vi "ObjectAvoid.vi"(7 "Stop?":bool, 8 "error in (no error)":errorcluster, 11 "RobotDriveDevRef":T1) -> (2 "Motor Values":dbl[](array[numeric]))   [LabVIEW 2015]
uses:
  <vilib>/Rock Robotics/WPI/RobotDrive/WPI_RobotDriveDevRef.ctl
  <vilib>/Rock Robotics/WPI/MotorControl/WPI_MotorControlDeviceRef.ctl
  <vilib>/Rock Robotics/WPI/MotorControl/WPI_MotorControlType.ctl
  <vilib>/Rock Robotics/SystemInterfaces/DIO/FPGA_DIOPWMChannel.ctl
  <vilib>/Rock Robotics/WPI/PWM/WPI_PWMDeadband.ctl
  <vilib>/Rock Robotics/WPI/CAN/Jaguar/SubVIs/WPI_CANJaguar_ControlMode.ctl
  <vilib>/Rock Robotics/WPI/CAN/TalonSRX/WPI_CANTalonSRX_APIControlMode.ctl
  Robot Global Data.vi
  <vilib>/Rock Robotics/WPI/RobotDrive/WPI_RobotDriveArcadeDrive_Standard(NoSaturation).vi
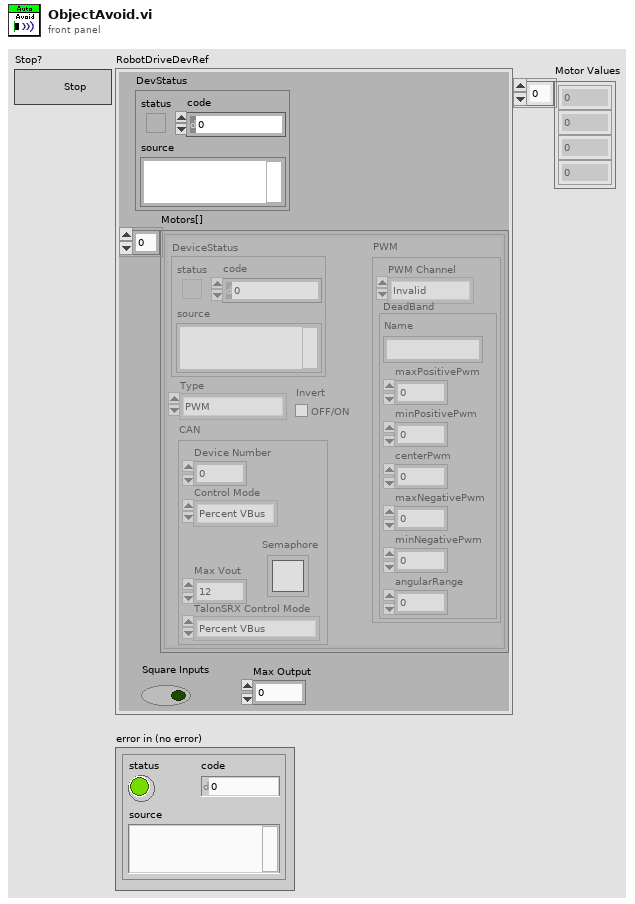
[diagram p1: front panel]
types:
  T1 = typedef "WPI_RobotDriveDevRef.ctl" = cluster{"DevStatus":errorcluster, "Motors[]":T2[], "Square Inputs":bool, "Max Output":dbl}
  T2 = typedef "WPI_MotorControlDeviceRef.ctl" = cluster{"DeviceStatus":errorcluster, "Type":T3, "PWM":cluster{"PWM Channel":T4, "DeadBand":T5}, "CAN":cluster{"Device Number":u8, "Control Mode":T6, "Semaphore":T7, "Max Vout":dbl, "TalonSRX Control Mode":T8}, "Invert":bool}
  T3 = typedef "WPI_MotorControlType.ctl" = enum16{"PWM", "CAN", "CANTalonSRX"}
  T4 = typedef "FPGA_DIOPWMChannel.ctl" = enum8{"PWM 0", "PWM 1", "PWM 2", "PWM 3", "PWM 4", "PWM 5", "PWM 6", "PWM 7", "PWM 8", "PWM 9", "PWM MXP 0", "PWM MXP 1", "PWM MXP 2", "PWM MXP 3", "PWM MXP 4", "PWM MXP 5", "PWM MXP 6", "PWM MXP 7", "PWM MXP 8", "PWM MXP 9", "Invalid"}
  T5 = typedef "WPI_PWMDeadband.ctl" = cluster{"Name":string, "maxPositivePwm":i32, "minPositivePwm":i32, "centerPwm":i32, "maxNegativePwm":i32, "minNegativePwm":i32, "angularRange":u16}
  T6 = typedef "WPI_CANJaguar_ControlMode.ctl" = enum8{"Percent VBus", "Current", "Speed", "Position", "Voltage"}
  T7 = typedef "Semaphore RefNum" = refnum<k1>
  T8 = typedef "WPI_CANTalonSRX_APIControlMode.ctl" = enum8{"Percent VBus", "Speed", "Position", "Slave", "Unchanged / Invalid", "Voltage Compensation", "Current", "Motion Profile"}
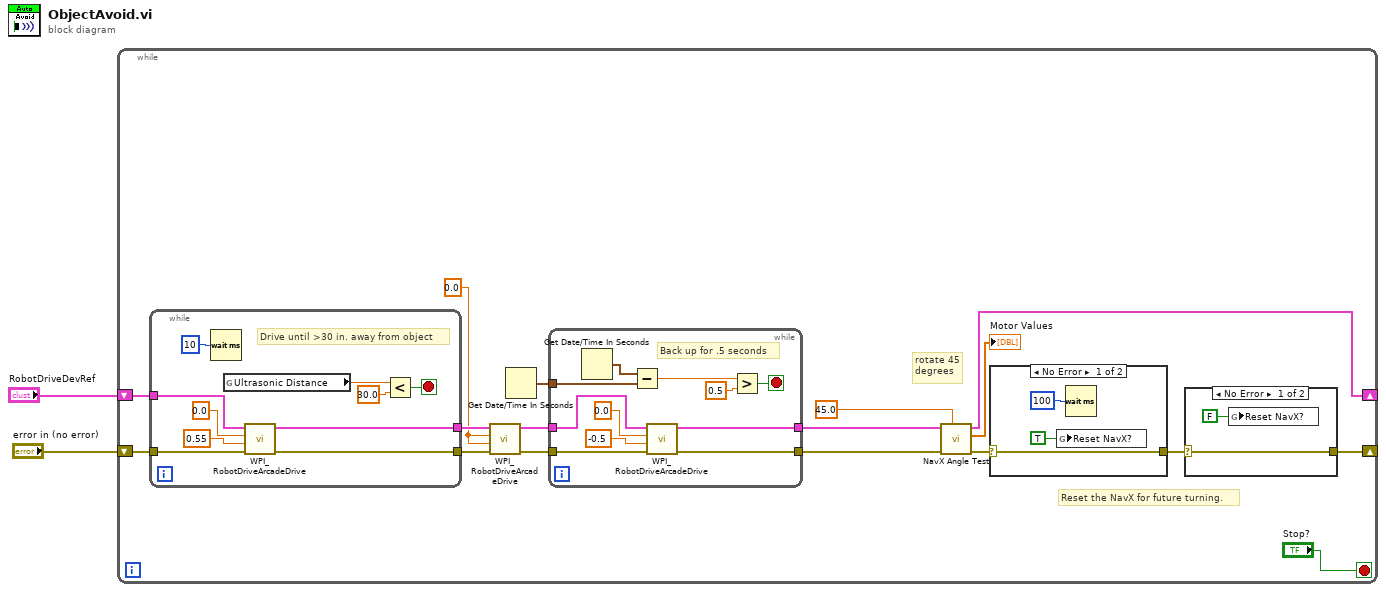
[diagram p0: block diagram]
diagram:
  n1 = while {
    shift-right: [w10] -> _
    shift-left: "RobotDriveDevRef" -> [w13]
    shift-right: [w6] -> _
    shift-left: "error in (no error)" -> [w5]
    stop <- "Stop?" stop-if-true
    w17 = 0.0 ("X axis value")
    # "Reset the NavX for future turning."
    # "rotate 45\ndegrees"
    n2 = while {
      tunnel: w13 -> [w43]
      tunnel: [w40] -> w19
      tunnel: [w39] -> w18
      tunnel: w5 -> [w38]
      stop <- w44 stop-if-true
      # "Drive until >30 in. away from object"
      n3 = Wait (ms)(milliseconds to wait=u32 10) -> ()  [unwired: 1 out]
      n4 = global read "Robot Global Data.vi" "Ultrasonic Distance"() -> (w46:dbl)
      n5 = call-poly <vilib>:"WPI_RobotDriveArcadeDrive.vi"("error in (no error)"=w38, "Y axis value"=0.55, "X axis value"=0.0, "RobotDriveDevRef"=w43) -> ("error out"=w39:errorcluster, "RobotDriveDevRef"=w40:T1)  [unwired: 5 in, 1 out]
      n6 = Less?(x=w46, y=30.0) -> (x < y?=w44:bool)
    }
    n7 = call-poly <vilib>:"WPI_RobotDriveArcadeDrive.vi"("error in (no error)"=w18, "Y axis value"=w17, "X axis value"=w17, "RobotDriveDevRef"=w19) -> ("error out"=w15:errorcluster, "RobotDriveDevRef"=w16:T1)  [unwired: 5 in, 1 out]
    n8 = Get Date/Time In Seconds() -> (seconds since 1Jan1904=w14:timestamp)
    n9 = while {
      tunnel: w16 -> [w37]
      tunnel: w15 -> [w36]
      tunnel: w14 -> [w31]
      tunnel: [w30] -> w12
      tunnel: [w29] -> w11
      stop <- w33 stop-if-true
      # "Back up for .5 seconds"
      n10 = Get Date/Time In Seconds() -> (seconds since 1Jan1904=w32:timestamp)
      n11 = Subtract(x=w32, y=w31) -> (x-y=w35:dbl)
      n12 = call-poly <vilib>:"WPI_RobotDriveArcadeDrive.vi"("error in (no error)"=w36, "Y axis value"=-0.5, "X axis value"=0.0, "RobotDriveDevRef"=w37) -> ("error out"=w29:errorcluster, "RobotDriveDevRef"=w30:T1)  [unwired: 5 in, 1 out]
      n13 = Greater?(x=w35, y=0.5) -> (0:w33:bool)
    }
    n14 = call "NavX Angle Test.vi"("Target Angle"=45.0, "Error In"=w11, "RobotDriveDevRefnum"=w12) -> ("error out"=w7:errorcluster, "Motor Values"=→"Motor Values":dbl[], "RobotDriveDevRef"=w10:T1)  [unwired: 6 in]
    n15 = case shown="No Error" w7 {
      selector: w7 -> [w25 w26]
      tunnel: [w25 w26] -> w8
      frame No Error {
        n16 = global write "Robot Global Data.vi" "Reset NavX?"(TRUE ("Reset NavX?")) -> ()
        n17 = Wait (ms)(milliseconds to wait=u32 100) -> ()  [unwired: 1 out]
      }
      frame Error {
      }
    }
    n18 = case shown="No Error" w8 {
      selector: w8 -> [w21 w22]
      tunnel: [w21 w22] -> w6
      frame No Error {
        n19 = global write "Robot Global Data.vi" "Reset NavX?"(FALSE ("Reset NavX?")) -> ()
      }
      frame Error {
      }
    }
  }
